vi "Video Frame to ROIed Frame.vi"(7 "Video Frame":refnum<class "Video Frame.lvclass">, 12 "ROI Descriptor":T1 {"Contours"."Type" items=["No Selection", "Point", "Line", "Rectangle", "Oval", "Polygon", "Freehand Region", "Annulus", "Unused2", "Unused3", "Broken Line", "Freehand Line", "Rotated Rectangle"]}, 13 "Apply? (T)":bool=TRUE) -> (8 "ROIed Video Frame":refnum<class "ROIed Video Frame.lvclass">)   [LabVIEW 2018, in "ROIed Video Frame.lvclass"]
uses:
  ROIed Video Frame.lvclass
  Video Frame/Video Frame.lvclass
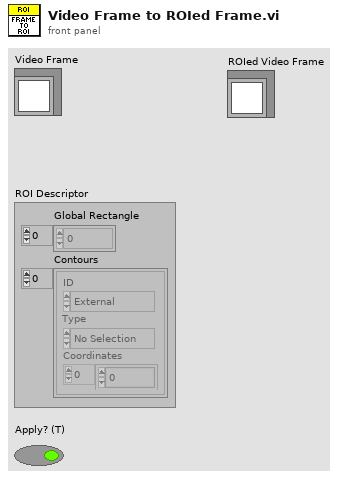
[diagram p1: front panel]
types:
  T1 = typedef "ROI Descriptor" = cluster{"Global Rectangle":i32[], "Contours":cluster{"ID":enum32{"External", "Internal"}, "Type":u32, "Coordinates":i32[]}[]}
  T2 = typedef "IMAQ Image.ctl" = refnum<image>
  T3 = cluster{"Width":u32, "Height":u32, "Frames Per Second":u32, "Codec":string, "Has Data":bool}
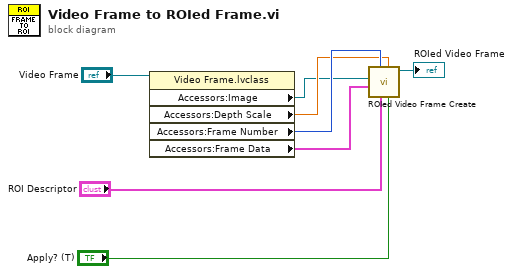
[diagram p0: block diagram]
diagram:
  n1 = property class="Video Frame.lvclass"(reference="Video Frame") -> ("Accessors:Image"=w2:T2, "Accessors:Depth Scale"=w3:dbl, "Accessors:Frame Number"=w4:i32, "Accessors:Frame Data"=w1:T3)  [unwired: 1 in, 2 out]
  n2 = call "ROIed Video Frame Create.vi"("Apply? (T)"="Apply? (T)", "Depth Scale"=w3, "ROI Descriptor"="ROI Descriptor", "Frame Number"=w4, "Frame Data"=w1, "Image Dst"=w2) -> ("ROIed Video Frame out"=→"ROIed Video Frame":refnum<class "ROIed Video Frame.lvclass">)  [unwired: 4 in, 1 out]
